vi "communication manager.vi"() -> ()   [LabVIEW 2018]
uses:
  communication-manager/socket SUB/socket SUB.lvclass
  C:/Users/Denis/Desktop/S4ACS/S4ACS/communication-manager/Socket/Socket.lvclass
  communication-manager/socket PUB/socket PUB.lvclass
  communication-manager/socket REP/socket REP.lvclass
  communication-manager/RxTx/CM_RxTx.lvclass
  <vilib>/addons/zeromq/zmq_context.lvclass
  communication-manager/Socket/Socket.lvclass
panel:
  in  "socket REP.lvclass":refnum<class "socket REP.lvclass">
  out "error out":errorcluster
  in  "socket PUB.lvclass":refnum<class "socket PUB.lvclass">
  in  "socket SUB.lvclass":refnum<class "socket SUB.lvclass">
  # "Communication Manager of S4CCS"
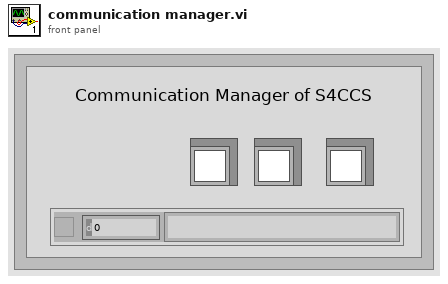
[diagram p1: front panel]
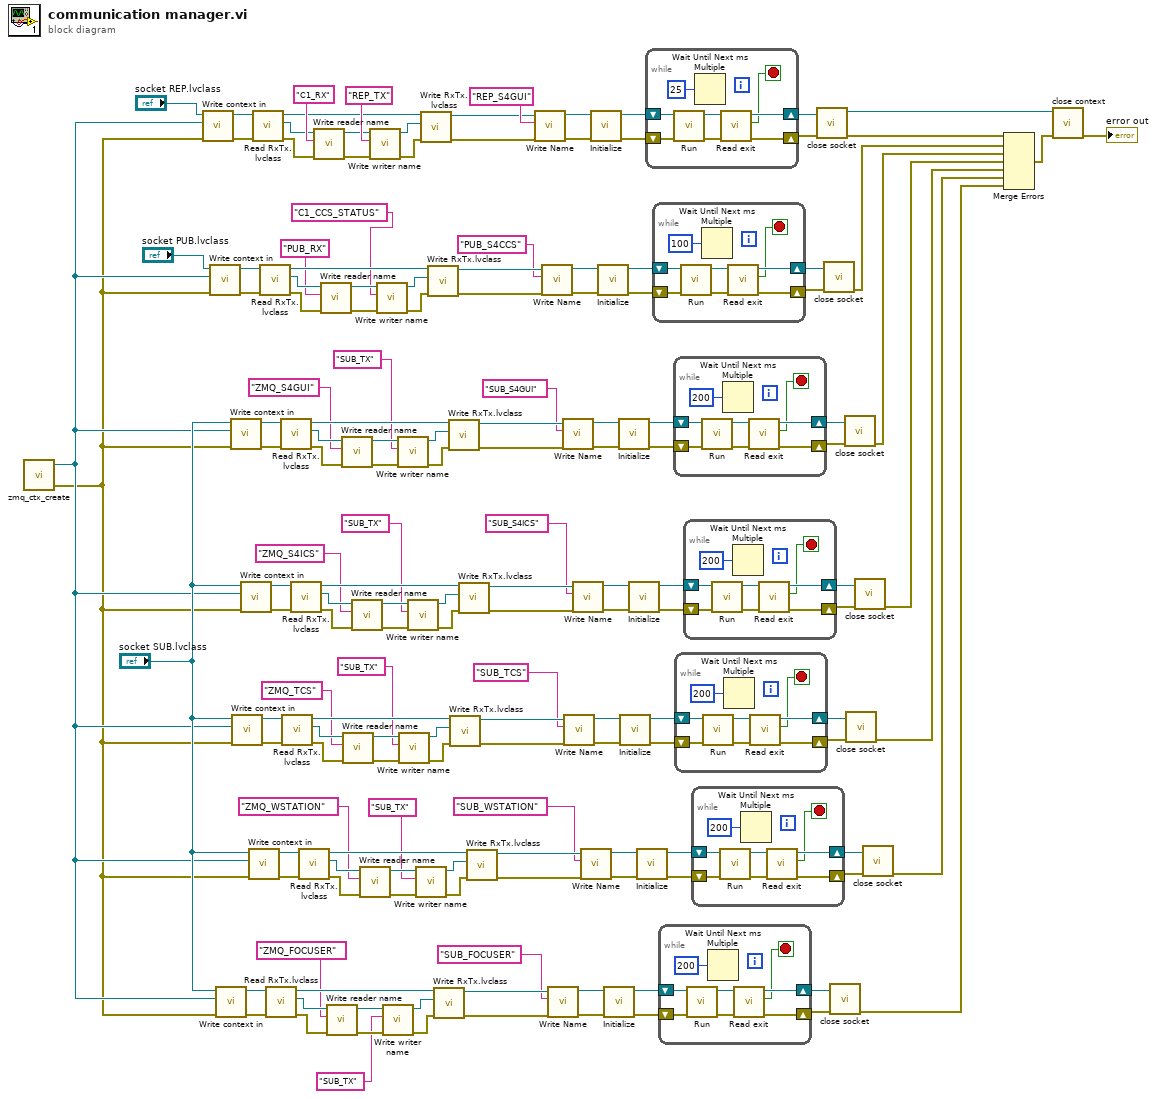
[diagram p0: block diagram]
diagram:
  n1 = call <vilib>:"zmq_ctx_create.vi"() -> ("error out"=w1:errorcluster, "context out"=w2:refnum<class "zmq_context.lvclass">)  [unwired: 4 in]
  n2 = call-dynamic "Write context in.vi"("error in (no error)"=w1, "zeromq.lvlib:ZeroMQ Context"=w2, "Socket in"="socket REP.lvclass") -> ("error out"=w132:errorcluster, "Socket out"=w133:refnum<class "socket REP.lvclass">)  [unwired: 7 in]
  n3 = call-dynamic "Write context in.vi"("error in (no error)"=w1, "zeromq.lvlib:ZeroMQ Context"=w2, "Socket in"="socket PUB.lvclass") -> ("error out"=w130:errorcluster, "Socket out"=w129:refnum<class "socket PUB.lvclass">)  [unwired: 7 in]
  n4 = call-dynamic "Write context in.vi"("error in (no error)"=w1, "zeromq.lvlib:ZeroMQ Context"=w2, "Socket in"="socket SUB.lvclass") -> ("error out"=w9:errorcluster, "Socket out"=w10:refnum<class "socket SUB.lvclass">)  [unwired: 7 in]
  n5 = call-dynamic "Write context in.vi"("error in (no error)"=w1, "zeromq.lvlib:ZeroMQ Context"=w2, "Socket in"="socket SUB.lvclass") -> ("error out"=w92:errorcluster, "Socket out"=w93:refnum<class "socket SUB.lvclass">)  [unwired: 7 in]
  n6 = call-dynamic "Write context in.vi"("error in (no error)"=w1, "zeromq.lvlib:ZeroMQ Context"=w2, "Socket in"="socket SUB.lvclass") -> ("error out"=w50:errorcluster, "Socket out"=w51:refnum<class "socket SUB.lvclass">)  [unwired: 7 in]
  n7 = call-dynamic "Write context in.vi"("error in (no error)"=w1, "zeromq.lvlib:ZeroMQ Context"=w2, "Socket in"="socket SUB.lvclass") -> ("error out"=w87:errorcluster, "Socket out"=w86:refnum<class "socket SUB.lvclass">)  [unwired: 7 in]
  n8 = call-dynamic "Write context in.vi"("error in (no error)"=w1, "zeromq.lvlib:ZeroMQ Context"=w2, "Socket in"="socket SUB.lvclass") -> ("error out"=w45:errorcluster, "Socket out"=w44:refnum<class "socket SUB.lvclass">)  [unwired: 7 in]
  n9 = call-dynamic "Read RxTx.lvclass.vi"("error in (no error)"=w132, "Socket in"=w133) -> ("error out"=w149:errorcluster, "RxTx.lvclass"=w153:refnum<class "CM_RxTx.lvclass">, "Socket out"=w150:refnum<class "socket REP.lvclass">)  [unwired: 7 in]
  n10 = call-dynamic "Read RxTx.lvclass.vi"("error in (no error)"=w130, "Socket in"=w129) -> ("error out"=w118:errorcluster, "RxTx.lvclass"=w114:refnum<class "CM_RxTx.lvclass">, "Socket out"=w117:refnum<class "socket PUB.lvclass">)  [unwired: 7 in]
  n11 = call-dynamic "Read RxTx.lvclass.vi"("error in (no error)"=w9, "Socket in"=w10) -> ("error out"=w21:errorcluster, "RxTx.lvclass"=w25:refnum<class "CM_RxTx.lvclass">, "Socket out"=w22:refnum<class "socket SUB.lvclass">)  [unwired: 7 in]
  n12 = call-dynamic "Read RxTx.lvclass.vi"("error in (no error)"=w92, "Socket in"=w93) -> ("error out"=w104:errorcluster, "RxTx.lvclass"=w108:refnum<class "CM_RxTx.lvclass">, "Socket out"=w105:refnum<class "socket SUB.lvclass">)  [unwired: 7 in]
  n13 = call-dynamic "Read RxTx.lvclass.vi"("error in (no error)"=w50, "Socket in"=w51) -> ("error out"=w62:errorcluster, "RxTx.lvclass"=w66:refnum<class "CM_RxTx.lvclass">, "Socket out"=w63:refnum<class "socket SUB.lvclass">)  [unwired: 7 in]
  n14 = call-dynamic "Read RxTx.lvclass.vi"("error in (no error)"=w87, "Socket in"=w86) -> ("error out"=w75:errorcluster, "RxTx.lvclass"=w71:refnum<class "CM_RxTx.lvclass">, "Socket out"=w74:refnum<class "socket SUB.lvclass">)  [unwired: 7 in]
  n15 = call-dynamic "Read RxTx.lvclass.vi"("error in (no error)"=w45, "Socket in"=w44) -> ("error out"=w33:errorcluster, "RxTx.lvclass"=w29:refnum<class "CM_RxTx.lvclass">, "Socket out"=w32:refnum<class "socket SUB.lvclass">)  [unwired: 7 in]
  n16 = call-dynamic "Write reader name.vi"("error in (no error)"=w149, "RX name"="C1_RX" ("reader name"), "RxTx in"=w153) -> ("error out"=w148:errorcluster, "RxTx out"=w152:refnum<class "CM_RxTx.lvclass">)  [unwired: 7 in]
  n17 = call-dynamic "Write reader name.vi"("error in (no error)"=w118, "RX name"="PUB_RX" ("reader name"), "RxTx in"=w114) -> ("error out"=w119:errorcluster, "RxTx out"=w115:refnum<class "CM_RxTx.lvclass">)  [unwired: 7 in]
  n18 = call-dynamic "Write reader name.vi"("error in (no error)"=w21, "RX name"="ZMQ_FOCUSER" ("reader name"), "RxTx in"=w25) -> ("error out"=w20:errorcluster, "RxTx out"=w24:refnum<class "CM_RxTx.lvclass">)  [unwired: 7 in]
  n19 = call-dynamic "Write reader name.vi"("error in (no error)"=w104, "RX name"="ZMQ_S4GUI" ("reader name"), "RxTx in"=w108) -> ("error out"=w103:errorcluster, "RxTx out"=w107:refnum<class "CM_RxTx.lvclass">)  [unwired: 7 in]
  n20 = call-dynamic "Write reader name.vi"("error in (no error)"=w62, "RX name"="ZMQ_TCS" ("reader name"), "RxTx in"=w66) -> ("error out"=w61:errorcluster, "RxTx out"=w65:refnum<class "CM_RxTx.lvclass">)  [unwired: 7 in]
  n21 = call-dynamic "Write reader name.vi"("error in (no error)"=w75, "RX name"="ZMQ_S4ICS" ("reader name"), "RxTx in"=w71) -> ("error out"=w76:errorcluster, "RxTx out"=w72:refnum<class "CM_RxTx.lvclass">)  [unwired: 7 in]
  n22 = call-dynamic "Write reader name.vi"("error in (no error)"=w33, "RX name"="ZMQ_WSTATION" ("reader name"), "RxTx in"=w29) -> ("error out"=w34:errorcluster, "RxTx out"=w30:refnum<class "CM_RxTx.lvclass">)  [unwired: 7 in]
  n23 = call-dynamic "Write writer name.vi"("error in (no error)"=w148, "Tx name"="REP_TX" ("writer name"), "RxTx in"=w152) -> ("error out"=w147:errorcluster, "RxTx out"=w151:refnum<class "CM_RxTx.lvclass">)  [unwired: 7 in]
  n24 = call-dynamic "Write writer name.vi"("error in (no error)"=w119, "Tx name"="C1_CCS_STATUS" ("writer name"), "RxTx in"=w115) -> ("error out"=w120:errorcluster, "RxTx out"=w116:refnum<class "CM_RxTx.lvclass">)  [unwired: 7 in]
  n25 = call-dynamic "Write writer name.vi"("error in (no error)"=w20, "Tx name"="SUB_TX" ("writer name"), "RxTx in"=w24) -> ("error out"=w19:errorcluster, "RxTx out"=w23:refnum<class "CM_RxTx.lvclass">)  [unwired: 7 in]
  n26 = call-dynamic "Write writer name.vi"("error in (no error)"=w103, "Tx name"="SUB_TX" ("writer name"), "RxTx in"=w107) -> ("error out"=w102:errorcluster, "RxTx out"=w106:refnum<class "CM_RxTx.lvclass">)  [unwired: 7 in]
  n27 = call-dynamic "Write writer name.vi"("error in (no error)"=w61, "Tx name"="SUB_TX" ("writer name"), "RxTx in"=w65) -> ("error out"=w60:errorcluster, "RxTx out"=w64:refnum<class "CM_RxTx.lvclass">)  [unwired: 7 in]
  n28 = call-dynamic "Write writer name.vi"("error in (no error)"=w76, "Tx name"="SUB_TX" ("writer name"), "RxTx in"=w72) -> ("error out"=w77:errorcluster, "RxTx out"=w73:refnum<class "CM_RxTx.lvclass">)  [unwired: 7 in]
  n29 = call-dynamic "Write writer name.vi"("error in (no error)"=w34, "Tx name"="SUB_TX" ("writer name"), "RxTx in"=w30) -> ("error out"=w35:errorcluster, "RxTx out"=w31:refnum<class "CM_RxTx.lvclass">)  [unwired: 7 in]
  n30 = call-dynamic "Write RxTx.lvclass.vi"("error in (no error)"=w147, "RxTx.lvclass"=w151, "Socket in"=w150) -> ("error out"=w144:errorcluster, "Socket out"=w145:refnum<class "socket REP.lvclass">)  [unwired: 7 in]
  n31 = call-dynamic "Write RxTx.lvclass.vi"("error in (no error)"=w120, "RxTx.lvclass"=w116, "Socket in"=w117) -> ("error out"=w122:errorcluster, "Socket out"=w121:refnum<class "socket PUB.lvclass">)  [unwired: 7 in]
  n32 = call-dynamic "Write RxTx.lvclass.vi"("error in (no error)"=w19, "RxTx.lvclass"=w23, "Socket in"=w22) -> ("error out"=w17:errorcluster, "Socket out"=w18:refnum<class "socket SUB.lvclass">)  [unwired: 7 in]
  n33 = call-dynamic "Write RxTx.lvclass.vi"("error in (no error)"=w102, "RxTx.lvclass"=w106, "Socket in"=w105) -> ("error out"=w100:errorcluster, "Socket out"=w101:refnum<class "socket SUB.lvclass">)  [unwired: 7 in]
  n34 = call-dynamic "Write RxTx.lvclass.vi"("error in (no error)"=w60, "RxTx.lvclass"=w64, "Socket in"=w63) -> ("error out"=w58:errorcluster, "Socket out"=w59:refnum<class "socket SUB.lvclass">)  [unwired: 7 in]
  n35 = call-dynamic "Write RxTx.lvclass.vi"("error in (no error)"=w77, "RxTx.lvclass"=w73, "Socket in"=w74) -> ("error out"=w79:errorcluster, "Socket out"=w78:refnum<class "socket SUB.lvclass">)  [unwired: 7 in]
  n36 = call-dynamic "Write RxTx.lvclass.vi"("error in (no error)"=w35, "RxTx.lvclass"=w31, "Socket in"=w32) -> ("error out"=w37:errorcluster, "Socket out"=w36:refnum<class "socket SUB.lvclass">)  [unwired: 7 in]
  n37 = call-dynamic "Write Name.vi"("error in (no error)"=w144, "Name"="REP_S4GUI", "Socket in"=w145) -> ("error out"=w134:errorcluster, "Socket out"=w135:refnum<class "socket REP.lvclass">)  [unwired: 7 in]
  n38 = call-dynamic "Write Name.vi"("error in (no error)"=w122, "Name"="PUB_S4CCS", "Socket in"=w121) -> ("error out"=w128:errorcluster, "Socket out"=w127:refnum<class "socket PUB.lvclass">)  [unwired: 7 in]
  n39 = call-dynamic "Write Name.vi"("error in (no error)"=w17, "Name"="SUB_FOCUSER", "Socket in"=w18) -> ("error out"=w11:errorcluster, "Socket out"=w12:refnum<class "socket SUB.lvclass">)  [unwired: 7 in]
  n40 = call-dynamic "Write Name.vi"("error in (no error)"=w100, "Name"="SUB_S4GUI", "Socket in"=w101) -> ("error out"=w94:errorcluster, "Socket out"=w95:refnum<class "socket SUB.lvclass">)  [unwired: 7 in]
  n41 = call-dynamic "Write Name.vi"("error in (no error)"=w58, "Name"="SUB_TCS", "Socket in"=w59) -> ("error out"=w52:errorcluster, "Socket out"=w53:refnum<class "socket SUB.lvclass">)  [unwired: 7 in]
  n42 = call-dynamic "Write Name.vi"("error in (no error)"=w79, "Name"="SUB_S4ICS", "Socket in"=w78) -> ("error out"=w85:errorcluster, "Socket out"=w84:refnum<class "socket SUB.lvclass">)  [unwired: 7 in]
  n43 = call-dynamic "Write Name.vi"("error in (no error)"=w37, "Name"="SUB_WSTATION", "Socket in"=w36) -> ("error out"=w43:errorcluster, "Socket out"=w42:refnum<class "socket SUB.lvclass">)  [unwired: 7 in]
  n44 = call-dynamic "Initialize.vi"("error in (no error)"=w134, "socket REP in"=w135) -> ("error out"=w141:errorcluster, "socket REP out"=w143:refnum<class "socket REP.lvclass">)  [unwired: 8 in]
  n45 = call-dynamic "Initialize.vi"("error in (no error)"=w128, "socket PUB in"=w127) -> ("error out"=w125:errorcluster, "socket PUB out"=w123:refnum<class "socket PUB.lvclass">)  [unwired: 8 in]
  n46 = call-dynamic "Initialize.vi"("error in (no error)"=w11, "socket SUB in"=w12) -> ("error out"=w14:errorcluster, "socket SUB out"=w16:refnum<class "socket SUB.lvclass">)  [unwired: 8 in]
  n47 = call-dynamic "Initialize.vi"("error in (no error)"=w94, "socket SUB in"=w95) -> ("error out"=w97:errorcluster, "socket SUB out"=w99:refnum<class "socket SUB.lvclass">)  [unwired: 8 in]
  n48 = call-dynamic "Initialize.vi"("error in (no error)"=w52, "socket SUB in"=w53) -> ("error out"=w55:errorcluster, "socket SUB out"=w57:refnum<class "socket SUB.lvclass">)  [unwired: 8 in]
  n49 = call-dynamic "Initialize.vi"("error in (no error)"=w85, "socket SUB in"=w84) -> ("error out"=w82:errorcluster, "socket SUB out"=w80:refnum<class "socket SUB.lvclass">)  [unwired: 8 in]
  n50 = call-dynamic "Initialize.vi"("error in (no error)"=w43, "socket SUB in"=w42) -> ("error out"=w40:errorcluster, "socket SUB out"=w38:refnum<class "socket SUB.lvclass">)  [unwired: 8 in]
  n51 = while {
    shift-right: [w161] -> w142
    shift-left: w143 -> [w163]
    shift-right: [w158] -> w140
    shift-left: w141 -> [w160]
    stop <- w157 stop-if-true
    n52 = call-dynamic "Run.vi"("error in (no error)"=w160, "socket REP in"=w163) -> ("error out"=w159:errorcluster, "socket REP out"=w162:refnum<class "socket REP.lvclass">)  [unwired: 8 in]
    n53 = Wait Until Next ms Multiple(millisecond multiple=u32 25) -> ()  [unwired: 1 out]
    n54 = call-dynamic "Read exit.vi"("error in (no error)"=w159, "Socket in"=w162) -> ("error out"=w158:errorcluster, "exit"=w157:bool, "Socket out"=w161:refnum<class "socket REP.lvclass">)  [unwired: 7 in]
  }
  n55 = while {
    shift-right: [w169] -> w124
    shift-left: w123 -> [w171]
    shift-right: [w166] -> w126
    shift-left: w125 -> [w168]
    stop <- w165 stop-if-true
    n56 = call-dynamic "Run.vi"("error in (no error)"=w168, "socket PUB in"=w171) -> ("error out"=w167:errorcluster, "socket PUB out"=w170:refnum<class "socket PUB.lvclass">)  [unwired: 8 in]
    n57 = Wait Until Next ms Multiple(millisecond multiple=u32 100) -> ()  [unwired: 1 out]
    n58 = call-dynamic "Read exit.vi"("error in (no error)"=w167, "Socket in"=w170) -> ("error out"=w166:errorcluster, "exit"=w165:bool, "Socket out"=w169:refnum<class "socket PUB.lvclass">)  [unwired: 7 in]
  }
  n59 = while {
    shift-right: [w177] -> w15
    shift-left: w16 -> [w179]
    shift-right: [w174] -> w13
    shift-left: w14 -> [w176]
    stop <- w173 stop-if-true
    n60 = call-dynamic "Run.vi"("error in (no error)"=w176, "socket SUB in"=w179) -> ("error out"=w175:errorcluster, "socket SUB out"=w178:refnum<class "socket SUB.lvclass">)  [unwired: 8 in]
    n61 = Wait Until Next ms Multiple(millisecond multiple=u32 200) -> ()  [unwired: 1 out]
    n62 = call-dynamic "Read exit.vi"("error in (no error)"=w175, "Socket in"=w178) -> ("error out"=w174:errorcluster, "exit"=w173:bool, "Socket out"=w177:refnum<class "socket SUB.lvclass">)  [unwired: 7 in]
  }
  n63 = while {
    shift-right: [w185] -> w98
    shift-left: w99 -> [w187]
    shift-right: [w182] -> w96
    shift-left: w97 -> [w184]
    stop <- w181 stop-if-true
    n64 = call-dynamic "Run.vi"("error in (no error)"=w184, "socket SUB in"=w187) -> ("error out"=w183:errorcluster, "socket SUB out"=w186:refnum<class "socket SUB.lvclass">)  [unwired: 8 in]
    n65 = Wait Until Next ms Multiple(millisecond multiple=u32 200) -> ()  [unwired: 1 out]
    n66 = call-dynamic "Read exit.vi"("error in (no error)"=w183, "Socket in"=w186) -> ("error out"=w182:errorcluster, "exit"=w181:bool, "Socket out"=w185:refnum<class "socket SUB.lvclass">)  [unwired: 7 in]
  }
  n67 = while {
    shift-right: [w193] -> w56
    shift-left: w57 -> [w195]
    shift-right: [w190] -> w54
    shift-left: w55 -> [w192]
    stop <- w189 stop-if-true
    n68 = call-dynamic "Run.vi"("error in (no error)"=w192, "socket SUB in"=w195) -> ("error out"=w191:errorcluster, "socket SUB out"=w194:refnum<class "socket SUB.lvclass">)  [unwired: 8 in]
    n69 = Wait Until Next ms Multiple(millisecond multiple=u32 200) -> ()  [unwired: 1 out]
    n70 = call-dynamic "Read exit.vi"("error in (no error)"=w191, "Socket in"=w194) -> ("error out"=w190:errorcluster, "exit"=w189:bool, "Socket out"=w193:refnum<class "socket SUB.lvclass">)  [unwired: 7 in]
  }
  n71 = while {
    shift-right: [w201] -> w81
    shift-left: w80 -> [w203]
    shift-right: [w198] -> w83
    shift-left: w82 -> [w200]
    stop <- w197 stop-if-true
    n72 = call-dynamic "Run.vi"("error in (no error)"=w200, "socket SUB in"=w203) -> ("error out"=w199:errorcluster, "socket SUB out"=w202:refnum<class "socket SUB.lvclass">)  [unwired: 8 in]
    n73 = Wait Until Next ms Multiple(millisecond multiple=u32 200) -> ()  [unwired: 1 out]
    n74 = call-dynamic "Read exit.vi"("error in (no error)"=w199, "Socket in"=w202) -> ("error out"=w198:errorcluster, "exit"=w197:bool, "Socket out"=w201:refnum<class "socket SUB.lvclass">)  [unwired: 7 in]
  }
  n75 = while {
    shift-right: [w209] -> w39
    shift-left: w38 -> [w211]
    shift-right: [w206] -> w41
    shift-left: w40 -> [w208]
    stop <- w205 stop-if-true
    n76 = call-dynamic "Run.vi"("error in (no error)"=w208, "socket SUB in"=w211) -> ("error out"=w207:errorcluster, "socket SUB out"=w210:refnum<class "socket SUB.lvclass">)  [unwired: 8 in]
    n77 = Wait Until Next ms Multiple(millisecond multiple=u32 200) -> ()  [unwired: 1 out]
    n78 = call-dynamic "Read exit.vi"("error in (no error)"=w207, "Socket in"=w210) -> ("error out"=w206:errorcluster, "exit"=w205:bool, "Socket out"=w209:refnum<class "socket SUB.lvclass">)  [unwired: 7 in]
  }
  n79 = call "close socket.vi"("error in (no error)"=w140, "Socket in"=w142) -> ("error out"=w139:errorcluster, "Socket out"=w137:refnum<class "socket REP.lvclass">)  [unwired: 8 in]
  n80 = call "close socket.vi"("error in (no error)"=w126, "Socket in"=w124) -> ("error out"=w110:errorcluster)  [unwired: 8 in, 1 out]
  n81 = call "close socket.vi"("error in (no error)"=w13, "Socket in"=w15) -> ("error out"=w7:errorcluster)  [unwired: 8 in, 1 out]
  n82 = call "close socket.vi"("error in (no error)"=w96, "Socket in"=w98) -> ("error out"=w88:errorcluster)  [unwired: 8 in, 1 out]
  n83 = call "close socket.vi"("error in (no error)"=w54, "Socket in"=w56) -> ("error out"=w46:errorcluster)  [unwired: 8 in, 1 out]
  n84 = call "close socket.vi"("error in (no error)"=w83, "Socket in"=w81) -> ("error out"=w67:errorcluster)  [unwired: 8 in, 1 out]
  n85 = call "close socket.vi"("error in (no error)"=w41, "Socket in"=w39) -> ("error out"=w8:errorcluster)  [unwired: 8 in, 1 out]
  n86 = Merge Errors(w139, w110, w88, w67, w46, w8, w7) -> (w138:errorcluster)
  n87 = call-dynamic "close context.vi"("error in (no error)"=w138, "Socket in"=w137) -> ("error out"=→"error out":errorcluster)  [unwired: 8 in, 1 out]
